vi "saveGeneral.vi"(0 "itemList":string[](array[string]), 5 "resultsStr":string[](array[string]), 7 "item":string[](array[string]), 9 "文件（使用对话框）":path, 11 "value":string[](array[string]), 12 "错误输入":errorcluster) -> (4 "NextTF":string, 6 "FextTF":string, 8 "cluResult":T1, 10 "endTimeTime":string caption="endTime", 15 "错误输出":errorcluster)   [LabVIEW 2011]
uses:
  dataType/cluResult.ctl
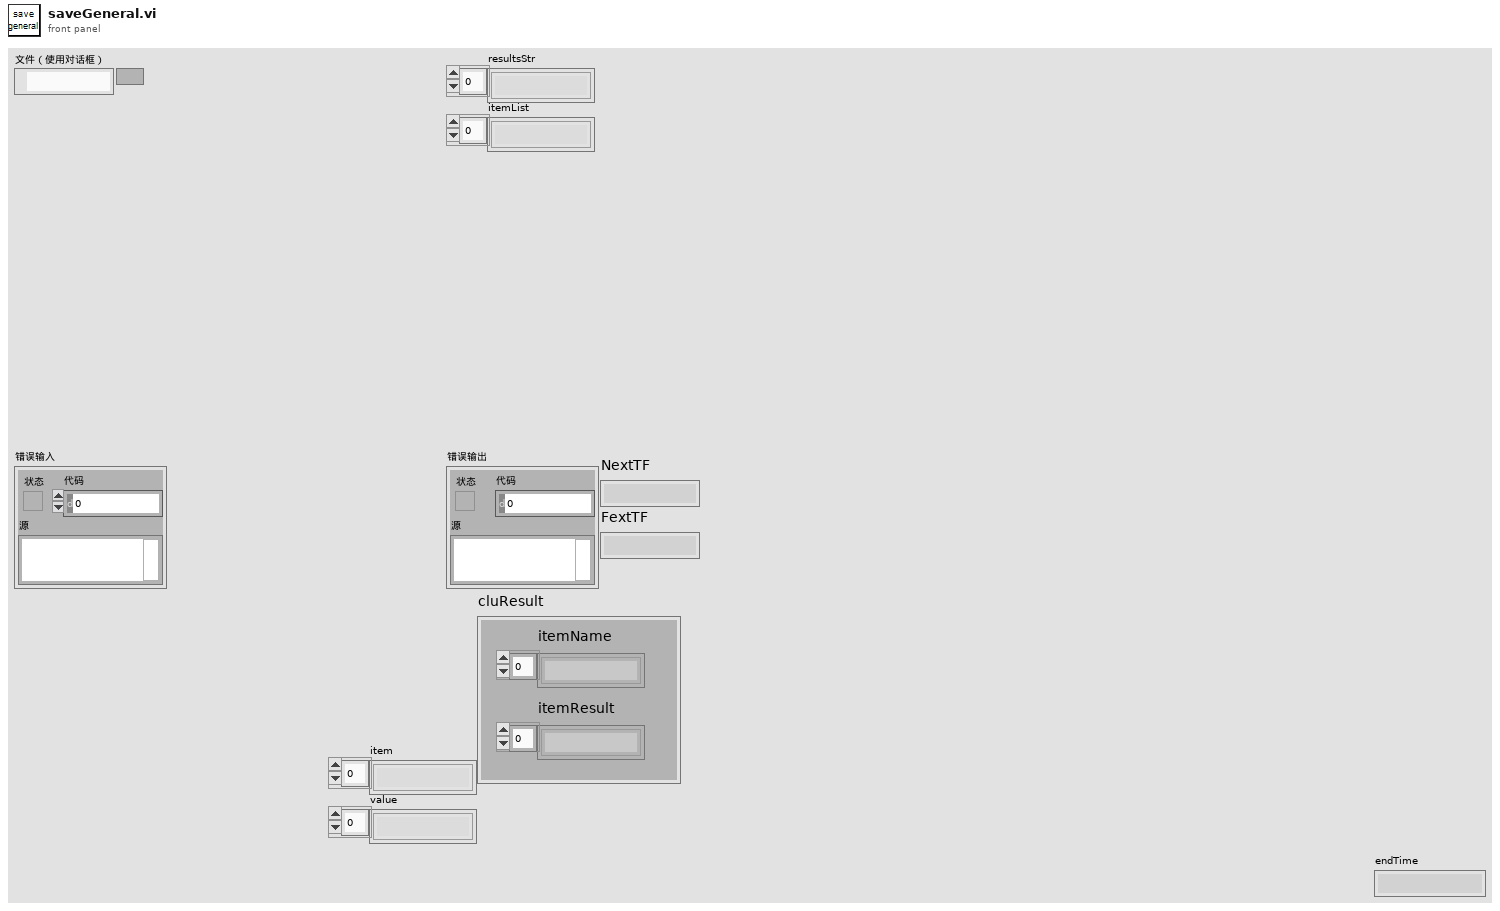
[diagram p1: front panel]
types:
  T1 = typedef "cluResult.ctl" = cluster{"itemResult":string[], "itemName":string[]}
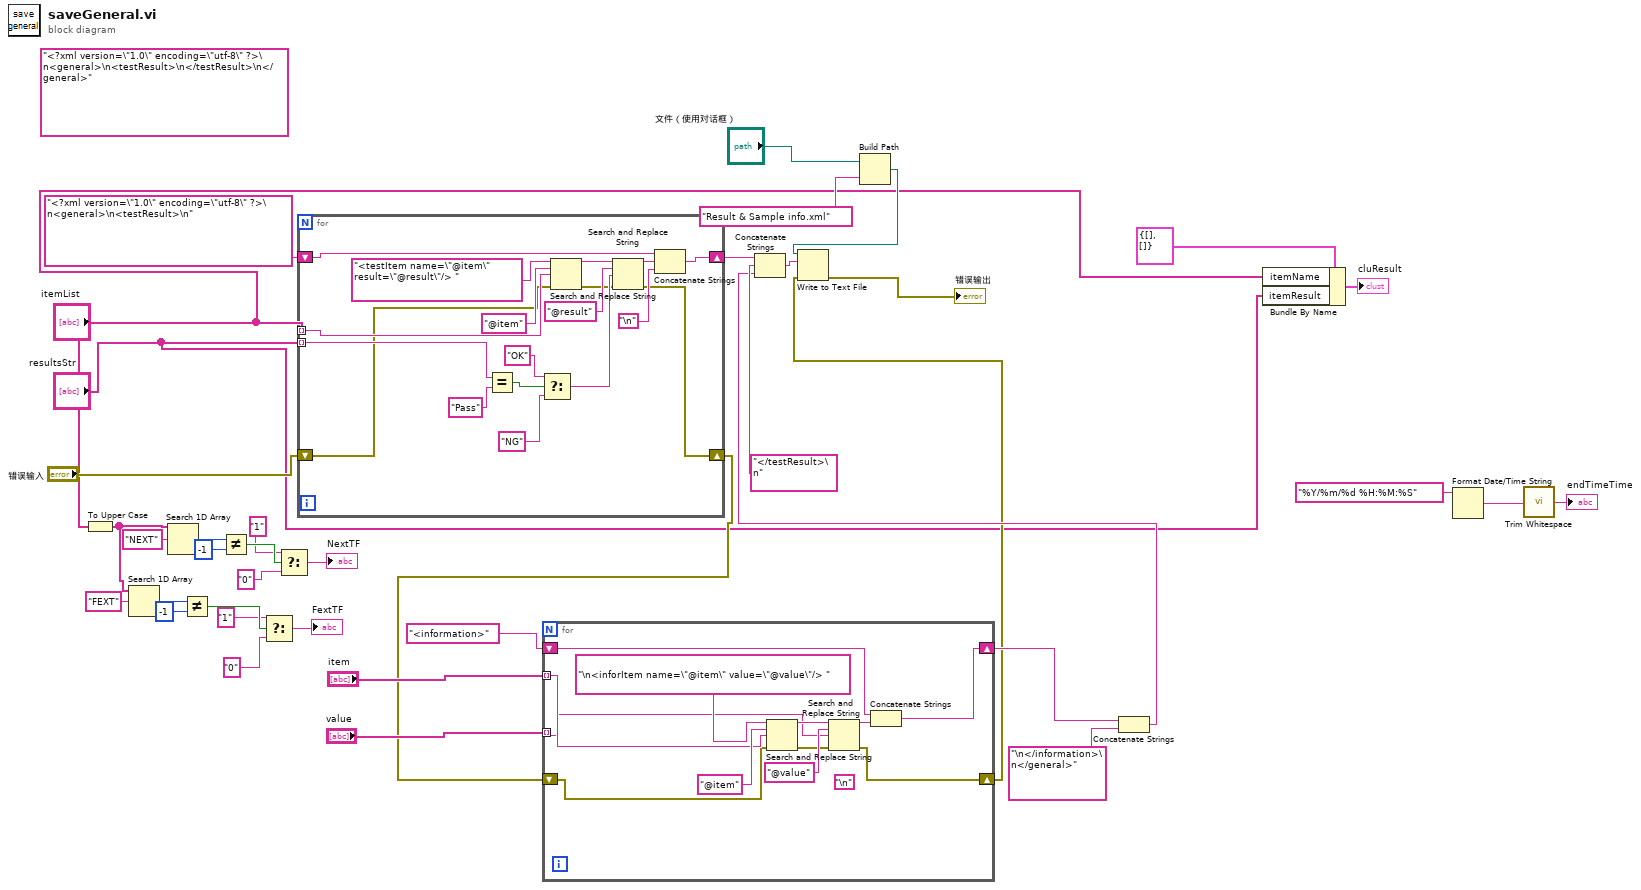
[diagram p0: block diagram]
diagram:
  (unwired) "<?xml version=\"1.0\" encoding=\"utf-8\" ?>\n<general>\n<testResult>\n</testResult>\n</general>"
  n1 = To Upper Case(1:"itemList") -> (0:w16:string[])
  n2 = Search 1D Array(1D array=w16, element="FEXT" ("元素")) -> (index of element=w18:i32)  [unwired: 1 in]
  n3 = Search 1D Array(1D array=w16, element="NEXT" ("元素")) -> (index of element=w21:i32)  [unwired: 1 in]
  n4 = Not Equal?(x=w18, y=-1) -> (x != y?=w14:bool)
  n5 = Not Equal?(x=w21, y=-1) -> (x != y?=w15:bool)
  n6 = Select(t="1", s=w14, f="0") -> (s? t:f=→"FextTF":string)
  n7 = Select(t="1", s=w15, f="0") -> (s? t:f=→"NextTF":string)
  n8 = for {
    tunnel: "itemList" -> [w55] mode=indexing
    tunnel: "resultsStr" -> [w48] mode=indexing
    shift-right: [w50] -> w38
    shift-left: "<?xml version=\"1.0\" encoding=\"utf-8\" ?>\n<general>\n<testResult>\n" -> [w51]
    shift-right: [w40] -> w25
    shift-left: "错误输入" -> [w42]
    n9 = Equal?(x=w48, y="Pass") -> (x = y?=w46:bool)
    n10 = Select(t="OK", s=w46, f="NG") -> (s? t:f=w43:string)
    n11 = Search and Replace String(input string="<testItem name=\"@item\" result=\"@result\"/> ", search string="@item" ("搜索字符串"), replace string=w55, error in=w42) -> (result string=w54:string, error out=w41:errorcluster)  [unwired: 4 in, 2 out]
    n12 = Search and Replace String(input string=w54, search string="@result" ("搜索字符串"), replace string=w43, error in=w41) -> (result string=w52:string, error out=w40:errorcluster)  [unwired: 4 in, 2 out]
    n13 = Concatenate Strings(w51, w52, "\n") -> (w50:string)
  }
  n14 = for {
    tunnel: "item" -> [w64] mode=indexing
    tunnel: "value" -> [w63] mode=indexing
    shift-right: [w61] -> w29
    shift-left: "<information>" -> [w62]
    shift-right: [w58] -> w24
    shift-left: w25 -> [w60]
    (unwired) "\n"
    n15 = Search and Replace String(input string="\n<inforItem name=\"@item\" value=\"@value\"/> ", search string="@item" ("搜索字符串"), replace string=w64, error in=w60) -> (result string=w68:string, error out=w59:errorcluster)  [unwired: 4 in, 2 out]
    n16 = Search and Replace String(input string=w68, search string="@value" ("搜索字符串"), replace string=w63, error in=w59) -> (result string=w66:string, error out=w58:errorcluster)  [unwired: 4 in, 2 out]
    n17 = Concatenate Strings(w62, w66) -> (w61:string)
  }
  n18 = Build Path(base path="文件（使用对话框）", name or relative path="Result & Sample info.xml" ("名称或相对路径")) -> (appended path=w33:path)
  n19 = Concatenate Strings(w29, "\n</information>\n</general>" ("字符串")) -> (w27:string)
  n20 = Concatenate Strings(w38, "</testResult>\n", w27) -> (w36:string)
  n21 = Write to Text File(file (use dialog)=w33, text=w36, error in=w24) -> (error out=→"错误输出":errorcluster)  [unwired: 1 in, 2 out]
  n22 = Bundle By Name(cluster=T1 {"itemResult"=[], "itemName"=[]} ("resultCluster"), "itemName"="itemList", "itemResult"="resultsStr") -> (→"cluResult":T1)
  n23 = Format Date/Time String(time format string (%c)="%Y/%m/%d %H:%M:%S" ("时间格式字符串(%c)")) -> (date/time string=w2:string)  [unwired: 2 in]
  n24 = call <vilib>:"Trim Whitespace.vi"("string"=w2) -> ("trimmed string"=→"endTimeTime":string)  [unwired: 1 in]
